vi "auto drive finished fg.vi"(1 "Done?":bool, 2 "Menu":T1) -> (0 "Done":bool)   [LabVIEW 2013]
uses:
  typedefs/fg_typedef.ctl
panel:
  # "Tell the auto state machine auto drive is done"
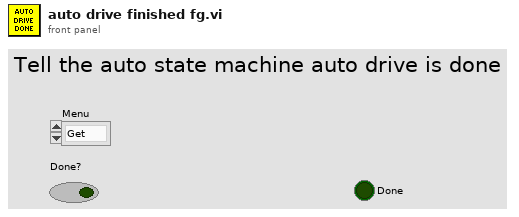
[diagram p1: front panel]
types:
  T1 = typedef "fg_typedef.ctl" = enum16{"Get", "Set"}
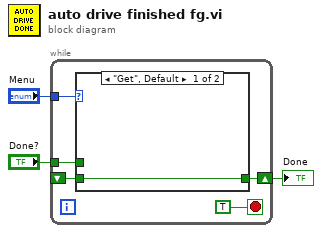
[diagram p0: block diagram]
diagram:
  n1 = while {
    shift-right: [w5] -> w1
    shift-left: _ -> [w4]
    tunnel: "Done?" -> [w8]
    tunnel: "Menu" -> [w7]
    stop <- TRUE stop-if-true
    n2 = case shown="\"Get\", Default" w7 {
      tunnel: w8 -> [_ w10]
      tunnel: [w9 w10] -> w5
      tunnel: w4 -> [w9 _]
      frame "Get", Default {
      }
      frame "Set" {
      }
    }
  }
  "Done" <- w1
